vi "pp3_trialTypes_isValid.vi"(0 "Trial Types In":T1[](array[typedef])=[{"Trial Type Number"=1, "Trial Type"=enum."GO", "Trial Weight"=1, "Shock (mA)"=-1.0, "Duration (ms)"=250.0, "Sound Type"=enum."04 FM Sweep", "Stim P1"=2000.0, "Stim P2"=4000.0, "Stim P3"=0.0, "Stim P4"=0.0, "DAQ Amplitude (V)"=1.0}, {"Trial Type Number"=2, "Trial Type"=enum."NOGO", "Trial Weight"=1, "Shock (mA)"=-1.0, "Duration (ms)"=250.0, "Sound Type"=enum."04 FM Sweep", "Stim P1"=4000.0, "Stim P2"=2000.0, "Stim P3"=0.0, "Stim P4"=0.0, "DAQ Amplitude (V)"=1.0}] {"DAQ Amplitude (V)" min=0.0 max=5.0 format="%_4g"; "Shock (mA)" min=-1.0 max=5.0; "Trial Weight" step=1; "Duration (ms)" min=0.0 max=1.0; "Trial Type Number" min=1 max=256 step=1}, 1 "Throw Error":bool, 5 "Total Trials":i32=60 min=2 step=2, 11 "error in (no error)":errorcluster) -> (3 "Trial Replication Factor":i32=30, 4 "Paradigm Valid?":bool=TRUE, 6 "GO Trials":T1[](array[typedef])=[{"Trial Type Number"=1, "Trial Type"=enum."GO", "Trial Weight"=1, "Shock (mA)"=-1.0, "Duration (ms)"=250.0, "Sound Type"=enum."04 FM Sweep", "Stim P1"=2000.0, "Stim P2"=4000.0, "Stim P3"=0.0, "Stim P4"=0.0, "DAQ Amplitude (V)"=1.0}] {"DAQ Amplitude (V)" min=0.0 max=5.0 format="%_4g"; "Shock (mA)" min=-1.0 max=5.0; "Trial Weight" step=1; "Duration (ms)" min=0.0 max=1.0; "Trial Type Number" min=1 max=256 step=1}, 8 "NOGO Trials":T1[](array[typedef])=[{"Trial Type Number"=2, "Trial Type"=enum."NOGO", "Trial Weight"=1, "Shock (mA)"=-1.0, "Duration (ms)"=250.0, "Sound Type"=enum."04 FM Sweep", "Stim P1"=4000.0, "Stim P2"=2000.0, "Stim P3"=0.0, "Stim P4"=0.0, "DAQ Amplitude (V)"=1.0}] {"DAQ Amplitude (V)" min=0.0 max=5.0 format="%_4g"; "Shock (mA)" min=-1.0 max=5.0; "Trial Weight" step=1; "Duration (ms)" min=0.0 max=1.0; "Trial Type Number" min=1 max=256 step=1}, 10 "TEST Trials":T1[](array[typedef]) {"DAQ Amplitude (V)" min=0.0 max=5.0 format="%_4g"; "Shock (mA)" min=-1.0 max=5.0; "Trial Weight" step=1; "Duration (ms)" min=0.0 max=1.0; "Trial Type Number" min=1 max=256 step=1}, 15 "error out":errorcluster)   [LabVIEW 2013]
uses:
  pp3_CTL_Trial.ctl
  pp3_CTL_TrialType.ctl
  labolabo2/waveforms/WFTypes.ctl
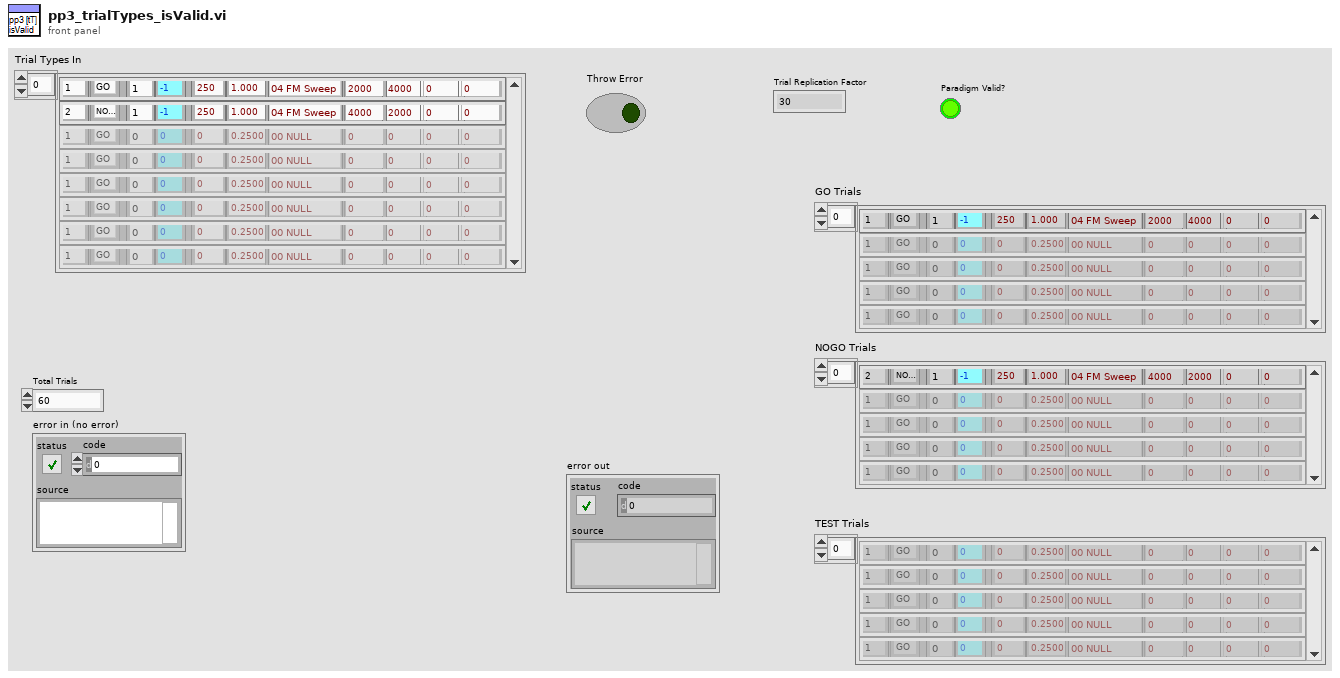
[diagram p1: front panel]
types:
  T1 = typedef "pp3_CTL_Trial.ctl" = cluster{"Trial Type Number":i16, "Trial Type":T2, "Trial Weight":u32, "Shock (mA)":dbl, "Duration (ms)":dbl, "Sound Type":T3, "Stim P1":dbl, "Stim P2":dbl, "Stim P3":dbl, "Stim P4":dbl, "DAQ Amplitude (V)":dbl}
  T2 = typedef "pp3_CTL_TrialType.ctl" = enum16{"OFF", "GO", "NOGO", "TEST"}
  T3 = typedef "WFTypes.ctl" = enum16{"00 NULL", "01 DC", "02 Noise", "03 Pure Tone", "04 FM Sweep"}
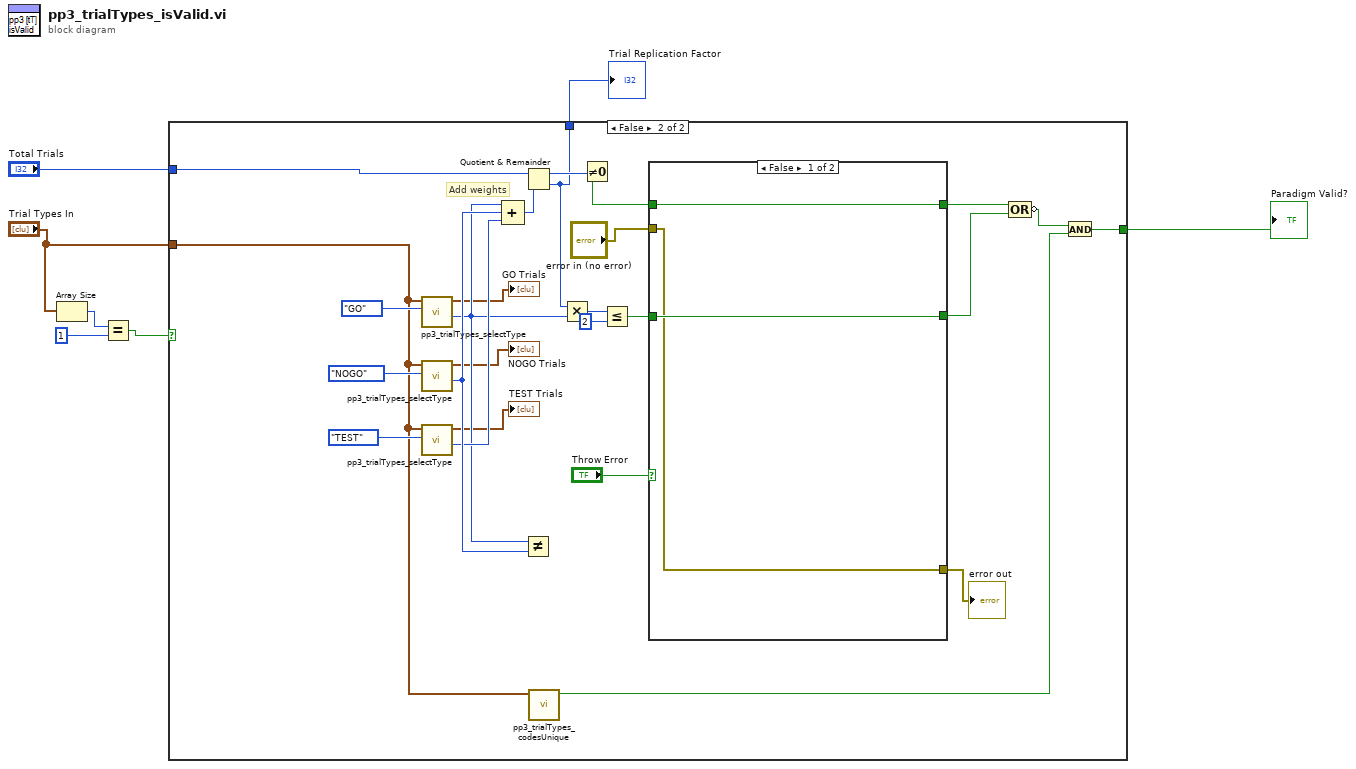
[diagram p0: block diagram]
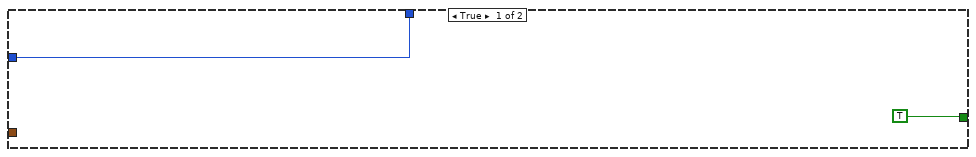
[diagram p2: hidden frame]
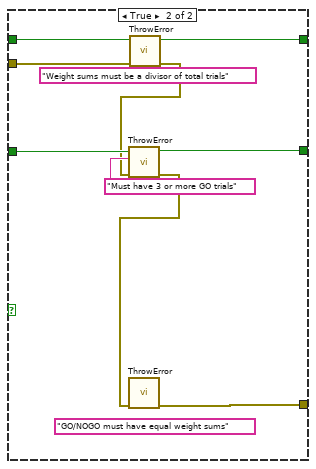
[diagram p3: hidden frame]
diagram:
  n1 = Array Size(array="Trial Types In") -> (size(s)=w3:i32)
  n2 = Equal?(x=w3, y=1) -> (x = y?=w1:bool)
  n3 = case shown="False" w1 {
    tunnel: "Total Trials" -> [w9 w27]
    tunnel: [TRUE w23] -> w6
    tunnel: [w9 w16] -> w5
    tunnel: "Trial Types In" -> [_ w13]
    frame True {
    }
    frame False {
      # "Add weights"
      n4 = call "pp3_trialTypes_selectType.vi"("Trial Type"=enum16{"OFF", "GO", "NOGO", "TEST"}."GO", "Trial Types In"=w13) -> ("Weight sums"=w14:u32, "Trial Types Out"=→"GO Trials":T1[])  [unwired: 7 in, 1 out]
      n5 = call "pp3_trialTypes_selectType.vi"("Trial Type"=enum16{"OFF", "GO", "NOGO", "TEST"}."NOGO", "Trial Types In"=w13) -> ("Weight sums"=w30:u32, "Trial Types Out"=→"NOGO Trials":T1[])  [unwired: 7 in, 1 out]
      n6 = call "pp3_trialTypes_selectType.vi"("Trial Type"=enum16{"OFF", "GO", "NOGO", "TEST"}."TEST", "Trial Types In"=w13) -> ("Weight sums"=w15:u32, "Trial Types Out"=→"TEST Trials":T1[])  [unwired: 7 in, 1 out]
      n7 = Compound Arithmetic op=ADD(w14, w30, w15) -> (w29:u32)
      n8 = Not Equal?(x=w14, y=w30) -> ()  [unwired: 1 out]
      n9 = Quotient & Remainder(x=w27, y=w29) -> (x-y*floor(x/y)=w18:u32, floor(x/y)=w16:u32)
      n10 = call "pp3_trialTypes_codesUnique.vi"("Trial Types"=w13) -> ("Codes unique?"=w19:bool)  [unwired: 9 in, 1 out]
      n11 = Multiply(x=w16, y=w14) -> (x*y=w17:u32)
      n12 = Not Equal To 0?(x=w18) -> (x != 0?=w28:bool)
      n13 = Less Or Equal?(x=w17, y=2) -> (x <= y?=w31:bool)
      n14 = case shown="False" "Throw Error" {
        tunnel: w31 -> [w37 w47]
        tunnel: w28 -> [w38 w45]
        tunnel: [w38 w42] -> w25
        tunnel: [w37 w41] -> w24
        tunnel: [w36 w40] -> w21
        tunnel: "error in (no error)" -> [w36 w39]
        frame False {
        }
        frame True {
          (unwired) "Weight sums must be a divisor of total trials" ("Error Message")
          (unwired) "GO/NOGO must have equal weight sums" ("Error Message")
          n15 = call "ThrowError.vi"("error in (no error)"=w39, "Error Input"=w45) -> ("error out"=w44:errorcluster, "Error Input Passthrough"=w42:bool)  [unwired: 8 in]
          n16 = call "ThrowError.vi"("error in (no error)"=w44, "Error Message"="Must have 3 or more GO trials", "Error Input"=w47) -> ("error out"=w43:errorcluster, "Error Input Passthrough"=w41:bool)  [unwired: 7 in]
          n17 = call "ThrowError.vi"("error in (no error)"=w43) -> ("error out"=w40:errorcluster)  [unwired: 9 in, 1 out]
        }
      }
      "error out" <- w21
      n18 = Compound Arithmetic op=OR(w25, w24) -> (invert w22:bool)
      n19 = And(x=w22, y=w19) -> (x .and. y?=w23:bool)
    }
  }
  "Paradigm Valid?" <- w6
  "Trial Replication Factor" <- w5
